vi "Create DAQ Data Waveform Structures.vi"(7 "Data Rate 9215 (S/s)":dbl=1200000.0 format="%#.6p", 8 "error in":errorcluster, 9 "Signal scaling":T1[](array[typedef]), 10 "RawDAQData in":T4, 11 "Data Rate 9775(S/s)":dbl=3.0 format="%#.6p") -> (0 "error out":errorcluster, 2 "InverterWaveforms":T2)   [LabVIEW 2019, in "Main.lvclass"]
doc: "Developed by Kevin Thompson\nkevin@thompsonengineering.net\n\nCopyright 2020\nThompson Engineering, LLC"
uses:
  Main.lvclass
  Common/DataTypes/RawDAQData--cluster.ctl
  Common/DataTypes/RawChannelData--cluster.ctl
  Common/DataTypes/InverterWaveforms--cluster.ctl
  Common/DataTypes/ChannelWaveforms--cluster.ctl
  subvis/DataTypes/Gain control.ctl
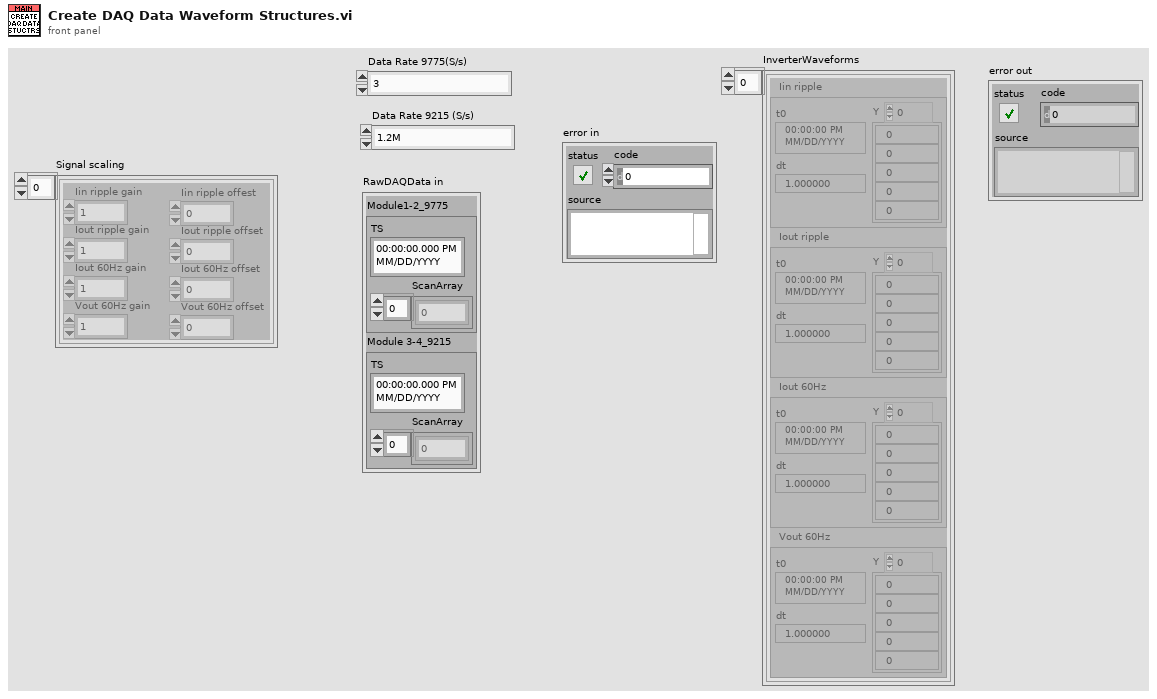
[diagram p1: front panel]
types:
  T1 = typedef "Main.lvclass/Gain control.ctl" = cluster{"Iin ripple gain":dbl, "Iout ripple gain":dbl, "Iout 60Hz gain ":dbl, "Vout 60Hz gain ":dbl, "Iin ripple offest":dbl, "Iout ripple offset":dbl, "Iout 60Hz offset":dbl, "Vout 60Hz offset":dbl}
  T2 = typedef "InverterWaveforms--cluster.ctl" = T3[]
  T3 = typedef "ChannelWaveforms--cluster.ctl" = cluster{"Iin ripple ":waveform(dbl), "Iout ripple ":waveform(dbl), "Iout 60Hz":waveform(dbl), "Vout 60Hz":waveform(dbl)}
  T4 = typedef "RawDAQData--cluster.ctl" = cluster{"Module1-2_9775":T5, "Module 3-4_9215":T5}
  T5 = typedef "RawChannelData--cluster.ctl" = cluster{"TS":timestamp, "ScanArray":dbl[]}
  T6 = cluster{"ch0":waveform(dbl), "ch1":waveform(dbl), "ch2":waveform(dbl), "ch3":waveform(dbl)}
  T7 = cluster{"ch0":waveform(dbl), "ch1":waveform(dbl), "ch2":waveform(dbl), "ch3":waveform(dbl)}[]
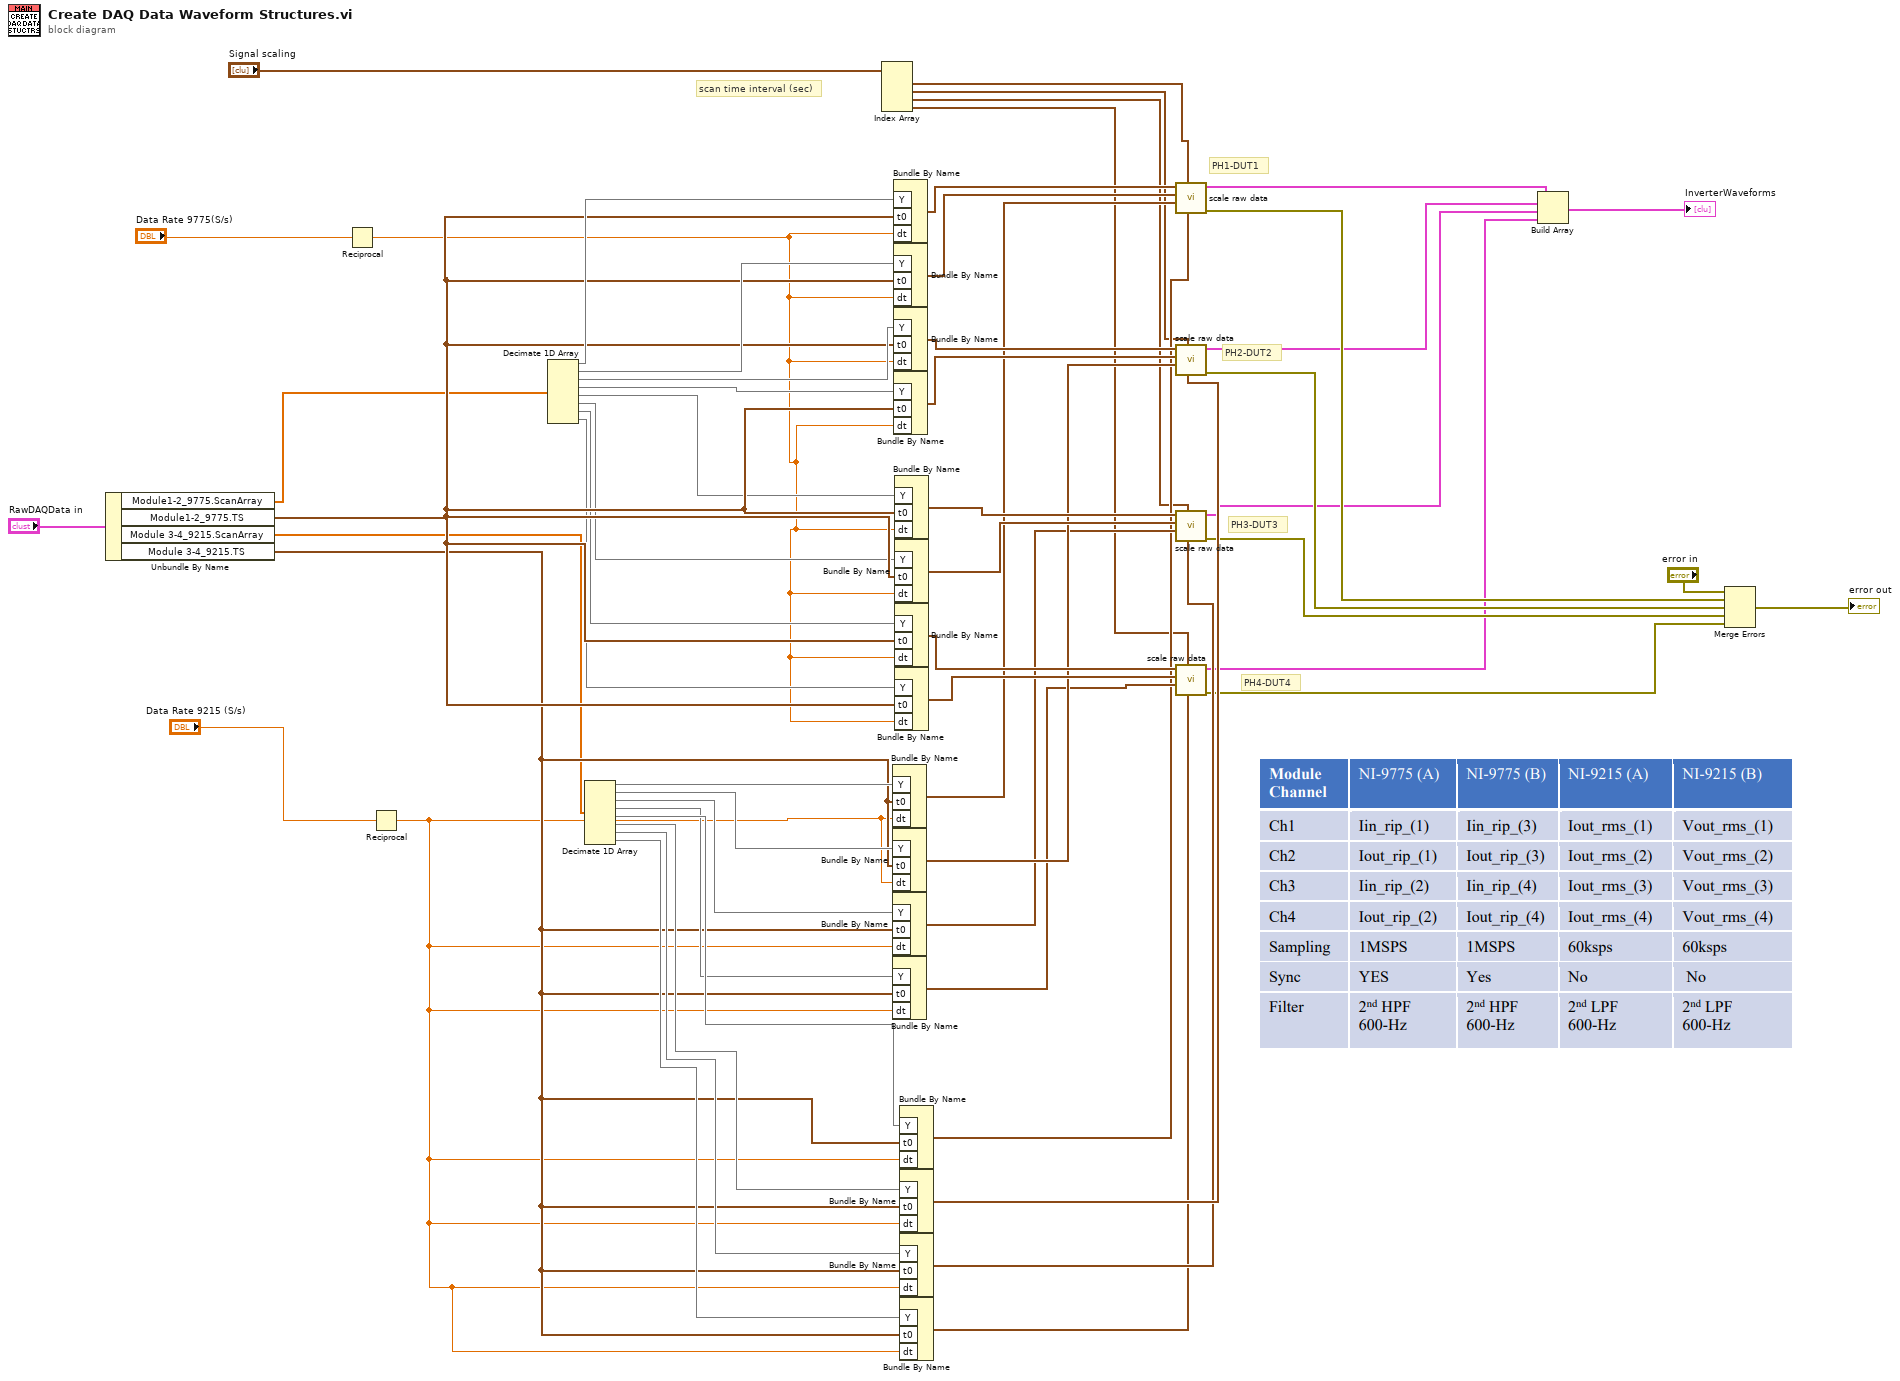
[diagram p0: block diagram]
diagram:
  # "PH4-DUT4"
  # "PH3-DUT3"
  # "PH2-DUT2"
  # "PH1-DUT1"
  # "scan time interval (sec)"
  n1 = Unbundle By Name("RawDAQData in") -> ("Module1-2_9775.ScanArray"=w37:dbl[], "Module1-2_9775.TS"=w52:timestamp, "Module 3-4_9215.ScanArray"=w38:dbl[], "Module 3-4_9215.TS"=w39:timestamp)
  n2 = Reciprocal(x="Data Rate 9775(S/s)") -> (1/x=w7:dbl)
  n3 = Reciprocal(x="Data Rate 9215 (S/s)") -> (1/x=w8:dbl)
  n4 = Decimate 1D Array(w37) -> (w56:dbl[], w55:dbl[], w54:dbl[], w53:dbl[], w51:dbl[], w50:dbl[], w49:dbl[], w48:dbl[])
  n5 = Decimate 1D Array(w38) -> (w40:dbl[], w41:dbl[], w42:dbl[], w43:dbl[], w44:dbl[], w45:dbl[], w46:dbl[], w47:dbl[])
  n6 = Index Array(array="Signal scaling") -> (element #1=w5:T1, element #2=w3:T1, element #3=w2:T1, element #4=w1:T1)  [unwired: 4 in]
  n7 = Bundle By Name("Y"=w40, "t0"=w39, "dt"=w8) -> (w28:waveform(dbl))  [unwired: 1 in]
  n8 = Bundle By Name("Y"=w41, "t0"=w39, "dt"=w8) -> (w27:waveform(dbl))  [unwired: 1 in]
  n9 = Bundle By Name("Y"=w42, "t0"=w39, "dt"=w8) -> (w26:waveform(dbl))  [unwired: 1 in]
  n10 = Bundle By Name("Y"=w43, "t0"=w39, "dt"=w8) -> (w25:waveform(dbl))  [unwired: 1 in]
  n11 = Bundle By Name("Y"=w56, "t0"=w52, "dt"=w7) -> (w36:waveform(dbl))  [unwired: 1 in]
  n12 = Bundle By Name("Y"=w55, "t0"=w52, "dt"=w7) -> (w35:waveform(dbl))  [unwired: 1 in]
  n13 = Bundle By Name("Y"=w54, "t0"=w52, "dt"=w7) -> (w34:waveform(dbl))  [unwired: 1 in]
  n14 = Bundle By Name("Y"=w53, "t0"=w52, "dt"=w7) -> (w33:waveform(dbl))  [unwired: 1 in]
  n15 = Bundle By Name("Y"=w51, "t0"=w52, "dt"=w7) -> (w32:waveform(dbl))  [unwired: 1 in]
  n16 = Bundle By Name("Y"=w50, "t0"=w52, "dt"=w7) -> (w31:waveform(dbl))  [unwired: 1 in]
  n17 = Bundle By Name("Y"=w49, "t0"=w52, "dt"=w7) -> (w30:waveform(dbl))  [unwired: 1 in]
  n18 = Bundle By Name("Y"=w48, "t0"=w52, "dt"=w7) -> (w29:waveform(dbl))  [unwired: 1 in]
  n19 = Bundle By Name("Y"=w44, "t0"=w39, "dt"=w8) -> (w24:waveform(dbl))  [unwired: 1 in]
  n20 = Bundle By Name("Y"=w45, "t0"=w39, "dt"=w8) -> (w23:waveform(dbl))  [unwired: 1 in]
  n21 = Bundle By Name("Y"=w46, "t0"=w39, "dt"=w8) -> (w22:waveform(dbl))  [unwired: 1 in]
  n22 = Bundle By Name("Y"=w47, "t0"=w39, "dt"=w8) -> (w21:waveform(dbl))  [unwired: 1 in]
  n23 = call "scale raw data.vi"("ch3"=w24, "Signal scaling control"=w5, "ch2"=w28, "ch1"=w35, "ch0"=w36) -> ("error out"=w19:errorcluster, "output channels WF"=w14:T6)  [unwired: 4 in, 1 out]
  n24 = call "scale raw data.vi"("ch3"=w23, "Signal scaling control"=w3, "ch2"=w27, "ch1"=w33, "ch0"=w34) -> ("error out"=w18:errorcluster, "output channels WF"=w13:T6)  [unwired: 4 in, 1 out]
  n25 = call "scale raw data.vi"("ch3"=w22, "Signal scaling control"=w2, "ch2"=w26, "ch1"=w31, "ch0"=w32) -> ("error out"=w17:errorcluster, "output channels WF"=w12:T6)  [unwired: 4 in, 1 out]
  n26 = call "scale raw data.vi"("ch3"=w21, "Signal scaling control"=w1, "ch2"=w25, "ch1"=w29, "ch0"=w30) -> ("error out"=w16:errorcluster, "output channels WF"=w11:T6)  [unwired: 4 in, 1 out]
  n27 = Build Array(w14, w13, w12, w11) -> (→"InverterWaveforms":T7)
  n28 = Merge Errors("error in", w19, w18, w17, w16) -> (→"error out":errorcluster)
